vi "Print Channel Values.vi"(8 "error in (no error)":errorcluster, 10 "Inputs?":bool, 11 "Channel Values":dbl[](array[numeric])) -> ()   [LabVIEW 2012, in "Shared Variable Custom Device.lvlib"]
uses:
  Shared Variable Custom Device.lvlib
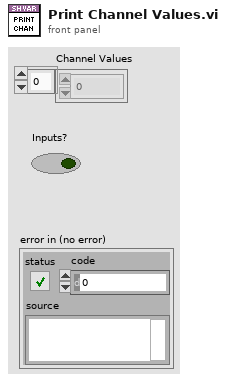
[diagram p1: front panel]
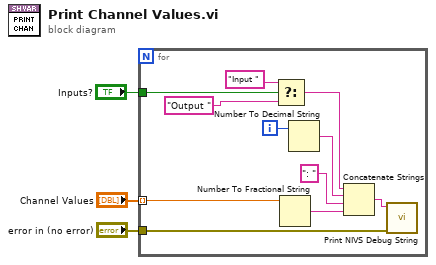
[diagram p0: block diagram]
diagram:
  n1 = for {
    tunnel: "error in (no error)" -> [w14]
    tunnel: "Channel Values" -> [w13] mode=indexing
    tunnel: "Inputs?" -> [w10]
    i -> [w6]
    n2 = Select(t="Input ", s=w10, f="Output ") -> (s? t:f=w7:string)
    n3 = Number To Fractional String(number=w13) -> (F-format string=w12:string)  [unwired: 3 in]
    n4 = Number To Decimal String(number=w6) -> (decimal integer string=w5:string)  [unwired: 1 in]
    n5 = Concatenate Strings(w7, w5, ": " ("string"), w12) -> (w11:string)
    n6 = call "Print NIVS Debug String.vi"("error in (no error)"=w14, "Debug String"=w11) -> ()  [unwired: 8 in, 1 out]
  }
